vi "ncs_voice.vi"() -> ()   [LabVIEW 2016]
uses:
  <instrlib>/niUSRP/niUSRP Timestamp.ctl
  <instrlib>/niUSRP/niUSRP Write Tx Data (2D CDB).vi
  <instrlib>/niUSRP/niUSRP Fetch Rx Data (2D CDB).vi
  <vilib>/Analysis/NI_AALBase.lvlib
  <vilib>/Analysis/3filter.llb/Filter Passband Type.ctl
  <vilib>/Analysis/baseanly.llb/IIR Cascade Filter (DBL).vi
panel:
  in  "Low-Pass Freq":dbl=10000.0 format="%#_13g"
  in  "Preset":string="v1a"
  out "Alarm":bool
  in  "Epsilon":dbl=0.05 format="%#_13g"
  in  "Timer":u16(ring)=90 items=["20min"=1200, "11min"=660, "10min"=600, "5.5min"=330, "2.5min"=150, "1.5min"=90]
  out "Elapsed Time (s)":dbl
  out "Time has Elapsed":bool
  in  "Timer Start":bool
  in  "File Name":string="freq2G_1"
  in  "Path":path=path "D:/Research/SummerFall17Spring18/CnC/NCS/Respiratory/BreathPattern_Cough_Speak/Data"
  out "NCS heartbeat":dbl[](graph)
  in  "Order":dbl=20.0 format="%#_13g"
  in  "High-Cutoff":dbl=8.0 format="%#_13g"
  in  "Low-Cutoff":dbl=0.5 format="%#_13g"
  out "size(s)":i32
  out "Coerced Rx IQ Rate":dbl
  in  "Sampling Rate":i32=20000
  out "Gain":dbl=-15.0
  out "Bandwidth":dbl=56000000.0
  out "Coerced Carrier Freq":dbl=2000000000.0 format="%#.17g"
  out "Coerced Tx IQ rate":dbl=1000000.0
  out "error IO":errorcluster={"status"=FALSE, "code"=-1074118647, "source"=""}
  in  "Rx #Samples":i32=20000
  in  "Tab Control 2":enum32{"NI-294x/295x", "NI-2900/2901"}(tab)=enum."NI-2900/2901"
  in  "Rx carrier frequency [Hz]":dbl=2000000000.0 format="%#_6p"
  in  "Tx carrier frequency [Hz]":dbl=1000000000.0 format="%#_6p"
  in  "Start Trigger Time":T1={"whole seconds"=1, "fractional seconds"=0.0}
  in  "Tab Control":T2(tab)
  out "NCS tag Amp":dbl[](graph)=[0.011967714738528729, 0.012021355192189592, 0.012015275039596582, 0.011969166030167903, 0.011958890166168242, 0.012007893820858737, 0.012022893722444085, 0.011978222225113794, 0.011969989939463181, 0.012003099640895068]
  out "NCS tag Phase":dbl[](graph)=[0.011967714738528729, 0.012021355192189592, 0.012015275039596582, 0.011969166030167903, 0.011958890166168242, 0.012007893820858737, 0.012022893722444085, 0.011978222225113794, 0.011969989939463181, 0.012003099640895068]
  out "Tag Amp":dbl[](graph)
  out "Tag Phase":dbl[](graph)
  out "Tx Waveform Graph":waveform(dbl)[](graph)
  in  "Stop":bool
  in  "Tone Amplitude":dbl=0.707 step=0.05 format="%#.6g"
  in  "Tone Frequency":dbl=10000.0 format="%#_6p"
  in  "Tx Waveform Size":dbl=200.0
  in  "Device Name":refnum<k15>="MyB210"
  in  "Tx Gain":dbl=28.0 format="%#_6f"
  in  "Tx IQ Rate":dbl=500000.0 format="%#_6p"
  in  "Rx Gain":dbl=32.0 format="%#_6f"
  in  "Rx IQ Rate":dbl=200000.0 format="%#_6p"
  # "Note that on the NI-2900 and NI-2901, both Rx channels share an LO and both Tx channels share an LO. However, on the NI-294x/295x devices, Rx and Tx of channel 0 share an LO and Rx and Tx of channel 1 share an LO."
  # "Rx Settings"
  # "Tx Settings"
  # "Channel 0"
  # "Heartbeat Filter"
  # "This Tx graph should always have end and start tied up since this is being sent in a loop continuously. Otherwise phase jumps will be noticed."
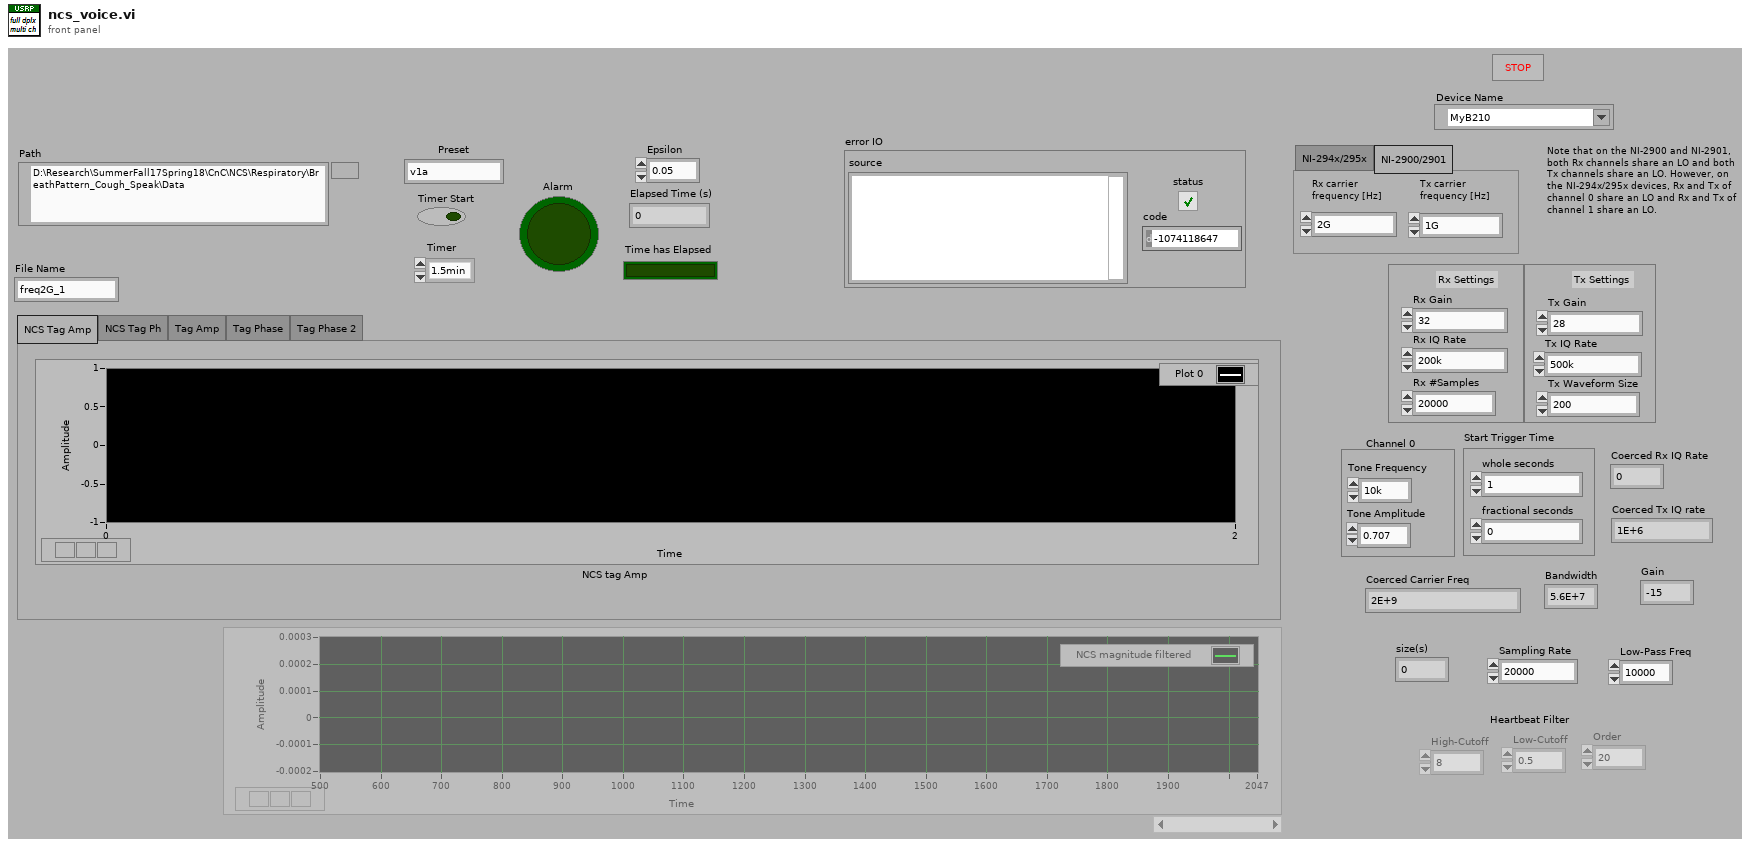
[diagram p1: front panel]
types:
  T1 = typedef "niUSRP Timestamp.ctl" = cluster{"whole seconds":u64, "fractional seconds":dbl}
  T2 = enum32{"NCS Tag Amp", "NCS Tag Ph", "Tag Amp", "Tag Phase", "Tag Phase 2"}
  T3 = typedef "NI_AALBase.lvlib/Filter Passband Type.ctl" = enum32{"Lowpass", "Highpass", "Bandpass", "Bandstop"}
  T4 = cluster{"filter structure":enum32{"IIR 2nd Order", "IIR 4th Order"}, "Reverse Coefficients":dbl[], "Forward Coefficients":dbl[]}
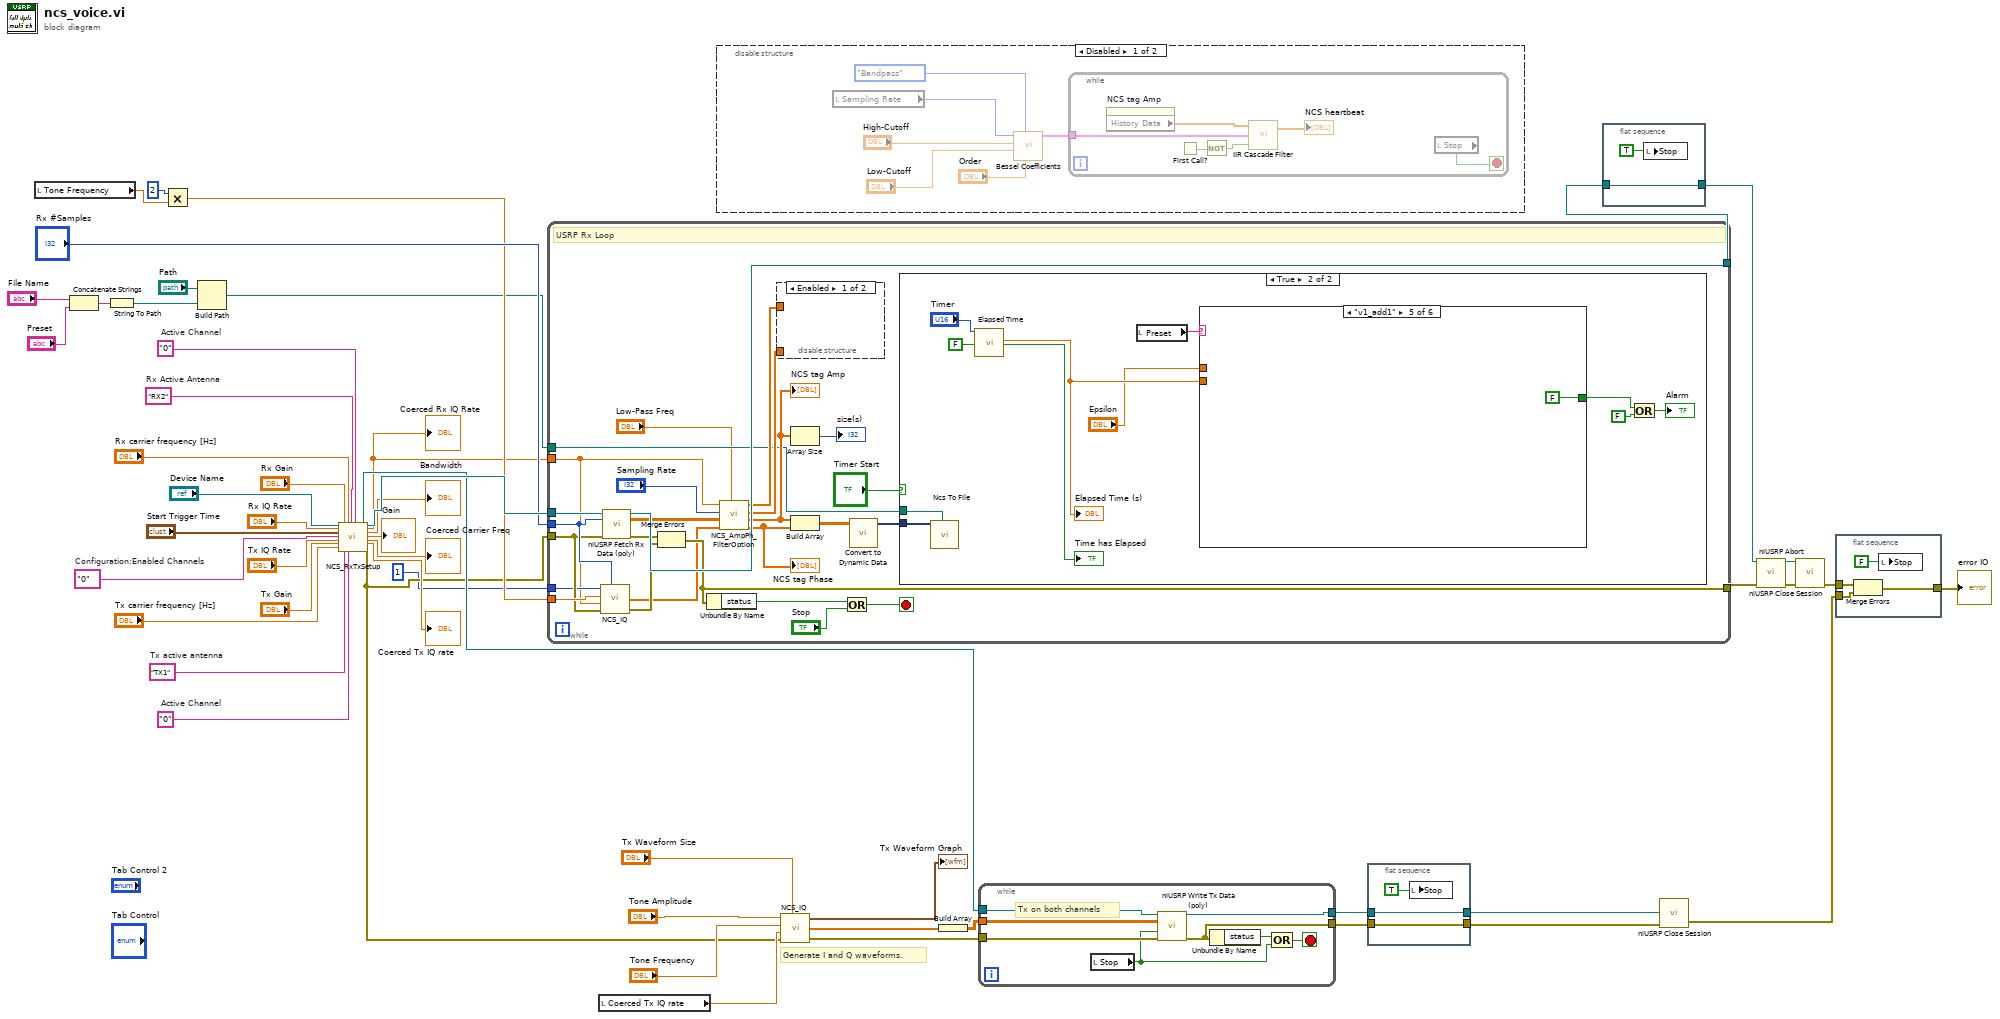
[diagram p0: block diagram]
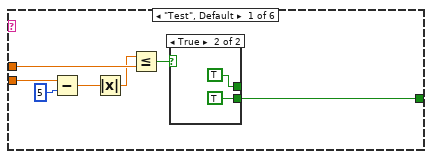
[diagram p4: hidden frame]
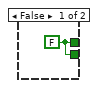
[diagram p5: hidden frame]
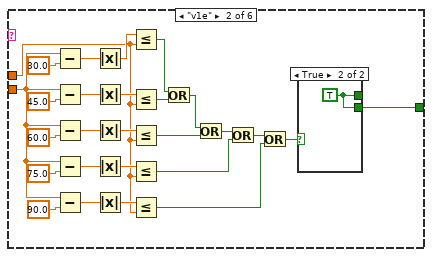
[diagram p6: hidden frame]
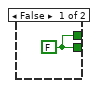
[diagram p7: hidden frame]
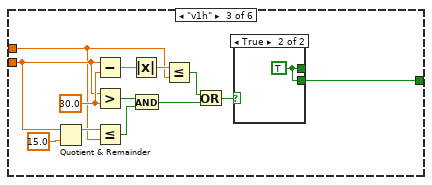
[diagram p8: hidden frame]
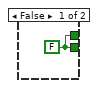
[diagram p9: hidden frame]
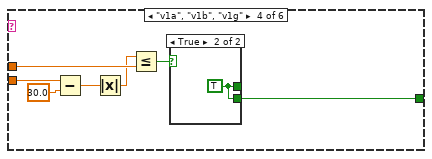
[diagram p10: hidden frame]
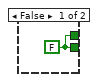
[diagram p11: hidden frame]
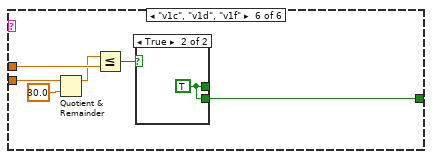
[diagram p12: hidden frame]
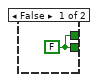
[diagram p13: hidden frame]
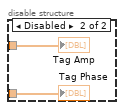
[diagram p14: hidden frame]
diagram:
  w8 = "0"  # Active Channel
  w9 = "0"  # Active Channel
  w44 = "RX2"  # Rx Active Antenna
  w40 = "TX1"  # Tx active antenna
  w26 = "0"  # Configuration:Enabled Channels
  # "Generate I and Q waveforms."
  n1 = local read "Tone Frequency"() -> (w25:dbl)
  n2 = Concatenate Strings("File Name", "Preset") -> (w2:string)
  n3 = String To Path(string=w2) -> (path=w6:path)
  n4 = Multiply(x=2, y=w25) -> (x*y=w24:dbl)
  n5 = Build Path(base path="Path", name or relative path=w6) -> (appended path=w4:path)
  n6 = call "NCS_RxTxSetup.vi"("IVI Refnum in"="Device Name", "Rx IQ Rate"="Rx IQ Rate", "Start Trigger Time"="Start Trigger Time", "Configuration:Enabled Channels"=w26, "Tx IQ Rate"="Tx IQ Rate", "Tx Gain"="Tx Gain", "Tx carrier frequency [Hz]"="Tx carrier frequency [Hz]", "Rx Gain"="Rx Gain", "Tx active antenna"=w40, "Rx carrier frequency [Hz]"="Rx carrier frequency [Hz]", "Active Channel"=w8, "Rx Active Antenna"=w44, "Active Channel 2"=w9) -> ("session handle out"=w51:refnum<k15>, "IVI Refnum out"=w52:refnum<k15>, "Coerced Rx IQ Rate"=w7:dbl, "Bandwidth"=→"Bandwidth":dbl, "Gain"=→"Gain":dbl, "Carrier Frequency"=→"Coerced Carrier Freq":dbl, "IQ Rate 2"=→"Coerced Tx IQ rate":dbl, "error out"=w19:errorcluster)  [unwired: 7 in]
  "Coerced Rx IQ Rate" <- w7
  n7 = while {
    tunnel: w52 -> [w78]
    tunnel: w19 -> [w70]
    tunnel: [w77] -> w36
    tunnel: "Rx #Samples" -> [w72]
    tunnel: w7 -> [w66]
    tunnel: [w67] -> w28
    tunnel: w24 -> [w71]
    tunnel: 1 -> [w68]
    tunnel: w4 -> [w56]
    stop <- w73 stop-if-true
    # "USRP Rx Loop"
    n8 = call "NCS_IQ.vi"("Tone Amplitude"=w68, "Waveform Size"=w72, "Tone Frequency"=w71, "Coerced IQ rate"=w66, "error in (no error)"=w70) -> ("IQ waveform array"=w64:cdb[], "error out"=w69:errorcluster)  [unwired: 1 in, 1 out]
    n9 = call-poly <instrlib>:"niUSRP Fetch Rx Data (poly).vi"("session handle"=w78, "number of samples"=w72, "error in (no error)"=w70) -> ("session handle out"=w77:refnum<k15>, "data"=w65:cdb[][], "error out"=w74:errorcluster)  [unwired: 9 in, 1 out]
    n10 = Merge Errors(w74, w69) -> (w67:errorcluster)
    n11 = Unbundle By Name(w67) -> ("status"=w76:bool)
    n12 = call "NCS_AmpPh_FilterOption.vi"("Low-Pass Freq"="Low-Pass Freq", "IQ"=w64, "data"=w65, "Sampling Rate"="Sampling Rate", "Coerced Rx IQ Rate"=w66) -> ("Phase DownSampled"=w57:dbl[], "Amp DownSampled"=w58:dbl[], "Unfiltered Phase"=w63:dbl[], "Unfiltered Amplitude"=w61:dbl[])  [unwired: 3 in]
    "NCS tag Amp" <- w58
    "NCS tag Phase" <- w57
    n13 = disable-structure shown="Enabled" {
      disable-tunnel: w61 -> [_ w163]
      disable-tunnel: w63 -> [_ w162]
      frame Enabled {
      }
      frame Disabled {
        "Tag Amp" <- w163
        "Tag Phase" <- w162
      }
    }
    n14 = Array Size(array=w58) -> (size(s)=→"size(s)":i32)
    n15 = Build Array(w58, w57) -> (w59:dbl[][])
    n16 = Or(x=w76, y="Stop") -> (x .or. y?=w73:bool)
    n17 = call "Convert to Dynamic Data"("2D Array"=w59) -> ("Dynamic Data Type"=w55:dynamicdata)  [unwired: 3 in]
    n18 = case shown="True" "Timer Start" {
      tunnel: w56 -> [_ w89]
      tunnel: w55 -> [_ w88]
      frame False {
      }
      frame True {
        n19 = call "Ncs To File"("Signals"=w88, "Filename"=w89) -> ()  [unwired: 15 in, 3 out]
        n20 = call "Elapsed Time"("Time Target (s)"="Timer", "Auto Reset"=FALSE) -> ("Elapsed Time (s)"=w84:dbl, "Time has Elapsed"=→"Time has Elapsed":bool)  [unwired: 10 in, 6 out]
        "Elapsed Time (s)" <- w84
        n21 = local read "Preset"() -> (w79:string)
        n22 = case shown="\"v1_add1\"" w79 {
          tunnel: w84 -> [w96 w107 w135 w148 _ w157]
          tunnel: "Epsilon" -> [w93 w101 w132 w147 _ w156]
          tunnel: [w92 w115 w138 w149 FALSE w158] -> w81
          frame "Test", Default {
            n23 = Subtract(x=w96, y=5) -> (x-y=w94:dbl)
            n24 = Absolute Value(x=w94) -> (abs(x)=w91:dbl)
            n25 = Less Or Equal?(x=w91, y=w93) -> (x <= y?=w90:bool)
            n26 = case shown="True" w90 {
              tunnel: [w97 TRUE] -> w92
              tunnel: [w97 TRUE] -> _
              frame False {
                w97 = FALSE
              }
              frame True {
              }
            }
          }
          frame "v1e" {
            n27 = Subtract(x=w107, y=30.0) -> (x-y=w125:dbl)
            n28 = Subtract(x=w107, y=45.0) -> (x-y=w122:dbl)
            n29 = Subtract(x=w107, y=60.0) -> (x-y=w118:dbl)
            n30 = Subtract(x=w107, y=75.0) -> (x-y=w114:dbl)
            n31 = Subtract(x=w107, y=90.0) -> (x-y=w110:dbl)
            n32 = Absolute Value(x=w125) -> (abs(x)=w124:dbl)
            n33 = Absolute Value(x=w122) -> (abs(x)=w121:dbl)
            n34 = Absolute Value(x=w118) -> (abs(x)=w117:dbl)
            n35 = Absolute Value(x=w114) -> (abs(x)=w113:dbl)
            n36 = Absolute Value(x=w110) -> (abs(x)=w109:dbl)
            n37 = Less Or Equal?(x=w124, y=w101) -> (x <= y?=w123:bool)
            n38 = Less Or Equal?(x=w121, y=w101) -> (x <= y?=w119:bool)
            n39 = Less Or Equal?(x=w117, y=w101) -> (x <= y?=w106:bool)
            n40 = Less Or Equal?(x=w113, y=w101) -> (x <= y?=w104:bool)
            n41 = Less Or Equal?(x=w109, y=w101) -> (x <= y?=w102:bool)
            n42 = Or(x=w123, y=w119) -> (x .or. y?=w111:bool)
            n43 = Or(x=w111, y=w106) -> (x .or. y?=w105:bool)
            n44 = Or(x=w105, y=w104) -> (x .or. y?=w103:bool)
            n45 = Or(x=w103, y=w102) -> (x .or. y?=w100:bool)
            n46 = case shown="True" w100 {
              tunnel: [w127 w128] -> _
              tunnel: [w127 w128] -> w115
              frame False {
                w127 = FALSE
              }
              frame True {
                w128 = TRUE
              }
            }
          }
          frame "v1h" {
            w137 = 30.0 ("y")
            n47 = Quotient & Remainder(x=w135, y=15.0) -> (x-y*floor(x/y)=w133:dbl)  [unwired: 1 out]
            n48 = Subtract(x=w135, y=w137) -> (x-y=w141:dbl)
            n49 = Greater?(x=w135, y=w137) -> (0:w136:bool)
            n50 = Less Or Equal?(x=w133, y=w132) -> (x <= y?=w131:bool)
            n51 = Absolute Value(x=w141) -> (abs(x)=w140:dbl)
            n52 = And(x=w136, y=w131) -> (x .and. y?=w130:bool)
            n53 = Less Or Equal?(x=w140, y=w132) -> (x <= y?=w139:bool)
            n54 = Or(x=w139, y=w130) -> (x .or. y?=w129:bool)
            n55 = case shown="True" w129 {
              tunnel: [w142 w143] -> _
              tunnel: [w142 w143] -> w138
              frame False {
                w142 = FALSE
              }
              frame True {
                w143 = TRUE
              }
            }
          }
          frame "v1a", "v1b", "v1g" {
            n56 = Subtract(x=w148, y=30.0) -> (x-y=w145:dbl)
            n57 = Absolute Value(x=w145) -> (abs(x)=w144:dbl)
            n58 = Less Or Equal?(x=w144, y=w147) -> (x <= y?=w146:bool)
            n59 = case shown="True" w146 {
              tunnel: [w151 w152] -> _
              tunnel: [w151 w152] -> w149
              frame False {
                w151 = FALSE
              }
              frame True {
                w152 = TRUE
              }
            }
          }
          frame "v1_add1" {
          }
          frame "v1c", "v1d", "v1f" {
            n60 = Quotient & Remainder(x=w157, y=30.0) -> (x-y*floor(x/y)=w154:dbl)  [unwired: 1 out]
            n61 = Less Or Equal?(x=w154, y=w156) -> (x <= y?=w155:bool)
            n62 = case shown="True" w155 {
              tunnel: [w160 w161] -> _
              tunnel: [w160 w161] -> w158
              frame False {
                w160 = FALSE
              }
              frame True {
                w161 = TRUE
              }
            }
          }
        }
        n63 = Or(x=w81, y=FALSE) -> (x .or. y?=→"Alarm":bool)
      }
    }
  }
  n64 = local read "Coerced Tx IQ rate"() -> (w20:dbl)
  n65 = disable-structure shown="Disabled" {
    frame Disabled {
      n66 = local read "Sampling Rate"() -> (w168:i32)
      n67 = call <vilib>:"Bessel Coefficients.vi"("order"="Order", "filter type"=Filter_Passband_Type."Bandpass", "low cutoff freq: fl"="Low-Cutoff", "high cutoff freq: fh"="High-Cutoff", "sampling freq: fs"=w168) -> ("IIR Filter Cluster"=w164:T4)  [unwired: 5 in, 1 out]
      n68 = while {
        tunnel: w164 -> [w172]
        stop <- w174 stop-if-true
        n69 = property on="NCS tag Amp" class="WaveformChart (strict)"() -> ("History Data"=w173:dbl[])  [unwired: 2 in, 2 out]
        n70 = First Call?() -> (First Call?: T/F=w175:bool)
        n71 = Not(x=w175) -> (.not. x?=w171:bool)
        n72 = call-poly <vilib>:"IIR Cascade Filter.vi"("init/cont (init:F)"=w171, "IIR Filter Cluster"=w172, "X"=w173) -> ("Filtered X"=→"NCS heartbeat":dbl[])  [unwired: 1 out]
        n73 = local read "Stop"() -> (w174:bool)
      }
    }
    frame Enabled {
    }
  }
  n74 = call "NCS_IQ.vi"("Tone Amplitude"="Tone Amplitude", "Waveform Size"="Tx Waveform Size", "Tone Frequency"="Tone Frequency", "Coerced IQ rate"=w20, "error in (no error)"=w19) -> ("IQ waveform"=→"Tx Waveform Graph":waveform(dbl)[], "IQ waveform array"=w17:cdb[], "error out"=w18:errorcluster)  [unwired: 1 in]
  n75 = Build Array(w17) -> (w48:cdb[][])
  n76 = while {
    tunnel: w51 -> [w183]
    tunnel: w18 -> [w182]
    tunnel: [w180] -> w39
    tunnel: [w178] -> w34
    tunnel: w48 -> [w176]
    stop <- w179 stop-if-true
    # "Tx on both channels"
    n77 = local read "Stop"() -> (w177:bool)
    n78 = call-poly <instrlib>:"niUSRP Write Tx Data (poly).vi"("session handle"=w183, "data"=w176, "end of data?"=w177, "error in (no error)"=w182) -> ("session handle out"=w178:refnum<k15>, "error out"=w180:errorcluster)  [unwired: 10 in]
    n79 = Unbundle By Name(w180) -> ("status"=w181:bool)
    n80 = Compound Arithmetic op=OR(w181, w177) -> (w179:bool)
  }
  n81 = flat-sequence {
    tunnel: [w185] -> w38
    tunnel: w39 -> [w185]
    tunnel: [w184] -> w35
    tunnel: w34 -> [w184]
    frame #0 {
      n82 = local write "Stop"(TRUE ("STOP")) -> ()
    }
  }
  n83 = flat-sequence {
    tunnel: [w187] -> w37
    tunnel: w36 -> [w187]
    frame #0 {
      n84 = local write "Stop"(TRUE ("STOP")) -> ()
    }
  }
  n85 = call <instrlib>:"niUSRP Close Session.vi"("session handle"=w35, "error in (no error)"=w38) -> ("error out"=w33:errorcluster)  [unwired: 13 in]
  n86 = call <instrlib>:"niUSRP Abort.vi"("session handle"=w37, "error in (no error)"=w28) -> ("session handle out"=w50:refnum<k15>, "error out"=w49:errorcluster)  [unwired: 12 in]
  n87 = call <instrlib>:"niUSRP Close Session.vi"("session handle"=w50, "error in (no error)"=w49) -> ("error out"=w30:errorcluster)  [unwired: 13 in]
  n88 = flat-sequence {
    tunnel: w33 -> [w191]
    tunnel: [w190] -> w31
    tunnel: w30 -> [w189]
    frame #0 {
      n89 = Merge Errors(w189, w191) -> (w190:errorcluster)
      n90 = local write "Stop"(FALSE ("STOP")) -> ()
    }
  }
  "error IO" <- w31
